vi "Make Test Suite.vi"(8 "error in (no error)":errorcluster) -> (0 "error out":errorcluster, 3 "LUnit Test Suite V2 out":refnum<class "LUnit Test Suite.lvclass">)   [LabVIEW 2020, in "Test Runner Test.lvclass"]
uses:
  Test Runner Test.lvclass
  source/API/LUnit Test Suite/LUnit Test Suite.lvclass
  C:/git/astemes-lunit/source/Core/Runnable/Runnable.lvclass
  Test Doubles/Test Case Test Double Child/Light Test Case Double.lvclass
  C:/git/astemes-lunit/source/API/LUnit Test Case/LUnit Test Case.lvclass
  Test Doubles/Test Case Test Double/Test Case Test Double.lvclass
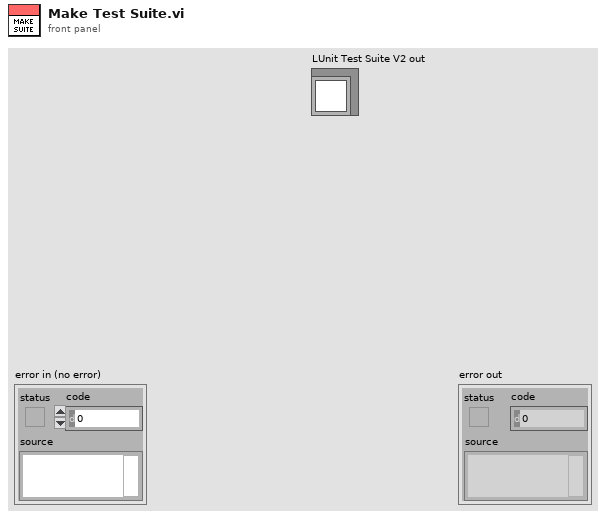
[diagram p1: front panel]
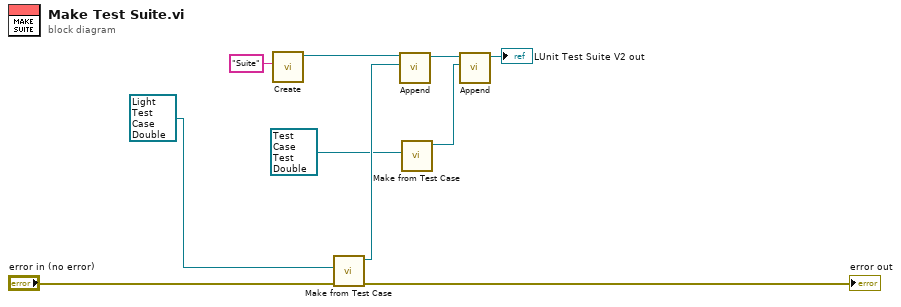
[diagram p0: block diagram]
diagram:
  n1 = call "Create.vi"("Suite Name"="Suite") -> ("LUnit Test Suite Out"=w7:refnum<class "LUnit Test Suite.lvclass">)  [unwired: 9 in, 1 out]
  n2 = call "Make from Test Case.vi"("error in (no error)"="error in (no error)", "LUnit Test Case"=refnum<class "Light Test Case Double.lvclass"> refnum ("Light Test Case Double.lvclass")) -> ("error out"=→"error out":errorcluster, "LUnit Test Suite Out"=w5:refnum<class "LUnit Test Suite.lvclass">)  [unwired: 8 in]
  n3 = call "Append.vi"("Runnable"=w5, "LUnit Test Suite In"=w7) -> ("LUnit Test Suite Out"=w4:refnum<class "LUnit Test Suite.lvclass">)  [unwired: 8 in, 1 out]
  n4 = call "Make from Test Case.vi"("LUnit Test Case"=refnum<class "Test Case Test Double.lvclass"> refnum ("Test Case Test Double.lvclass")) -> ("LUnit Test Suite Out"=w1:refnum<class "LUnit Test Suite.lvclass">)  [unwired: 9 in, 1 out]
  n5 = call "Append.vi"("Runnable"=w1, "LUnit Test Suite In"=w4) -> ("LUnit Test Suite Out"=→"LUnit Test Suite V2 out":refnum<class "LUnit Test Suite.lvclass">)  [unwired: 8 in, 1 out]
